vi "ActionVIOnCompile.vi"(8 "error in (no error)":errorcluster, 11 "Device Item Ref in":T1 format="%.0x") -> (0 "error out":errorcluster)   [LabVIEW 2016, in "UDP-Custom-Device System Explorer.lvlib"]
uses:
  UDP-Custom-Device System Explorer.lvlib
  <vilib>/NI Veristand/Custom Device API/Custom Device Item Ref.ctl
  Shared/Compiled.Settings.ctl
  Shared/Types/Shared - Rx.PacketInfo.ctl
  Shared/Types/Shared - Channel Data Type.ctl
  Shared/Types/Shared - Buffered.PacketInfo.ctl
  Shared/Types/Shared - Pointer Encoding.ctl
  Shared/Types/Shared - Receive Buffer Options.ctl
  Shared/Types/Shared - Transmit Buffer Options.ctl
  Shared/Types/Shared - Duplex Settings.ctl
  Shared/Types/Shared - New Data Options.ctl
  Shared/Types/Shared - Tx.PacketInfo.ctl
  Shared/Types/Shared - Transmit Flag Options.ctl
  Shared/Types/Shared - Transmit Echo Options.ctl
  Shared/Types/Shared - Transmit Sim Options.ctl
  Shared/Types/Shared - Header Details.ctl
  <vilib>/NI Veristand/Custom Device API/Set Item Property (Variant).vi
  <vilib>/NI VeriStand/Custom Device API/Custom Device API.lvlib
  <vilib>/NI/NIVS Inline Async API/_Data Access System Explorer/Data Access System Explorer.lvlib
  Shared/UDP-Custom-Device Shared.lvlib
panel:
  out "appended array":T2(array[cluster]) {"VS Refs" format="%.0x"}
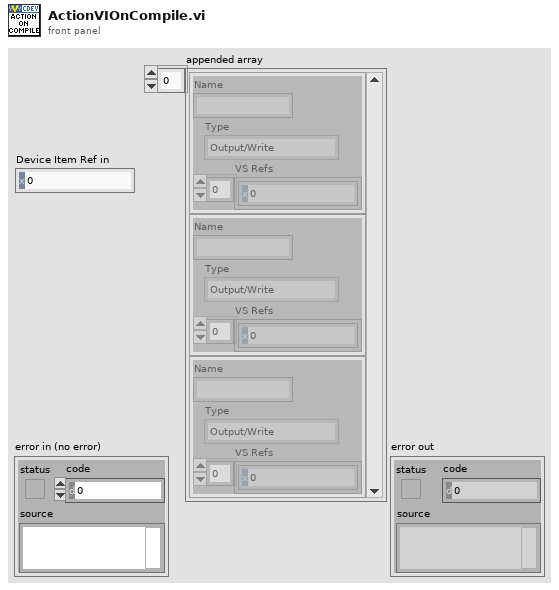
[diagram p1: front panel]
types:
  T1 = typedef "Custom Device API.lvlib/Custom Device Item Ref.ctl" = u64
  T2 = cluster{"Name":string, "Type":enum16{"Output/Write", "Input/Read", "Input/ReadWrite"}, "VS Refs":T1[]}[]
  T3 = typedef "UDP-Custom-Device Shared.lvlib/Compiled.Settings.ctl" = cluster{"Name":string, "Tx Enabled?":bool, "Rx Enabled?":bool, "Rx Packet Info":T4[], "Tx Packet Info":T11[], "Duplex Packets":refnum<data-value>}
  T4 = typedef "UDP-Custom-Device Shared.lvlib/Shared - Rx.PacketInfo.ctl" = cluster{"Packet Name":string, "Packet ID":i32, "Timeout":i32, "Rx IP Address":string, "Rx Port":u16, "Endianness":u16, "Multicast":bool, "Multicast IP Address":string, "Diagnostics En?":bool, "Debug Mode":bool, "Header Info":bool[], "Channel Data Types":T5[], "Buffered Packet Info":T6, "Duplex Packets":refnum<data-value>, "New Data Option":T10, "targetPriority":i16, "targetProcessor":i8}
  T5 = typedef "UDP-Custom-Device Shared.lvlib/Shared - Channel Data Type.ctl" = enum16{"Boolean", "Single", "Double", "I8", "I16", "I32", "I64", "U8", "U16", "U32", "U64"}
  T6 = typedef "UDP-Custom-Device Shared.lvlib/Shared - Buffered.PacketInfo.ctl" = cluster{"Buffer Size":i32, "External Buffer":bool, "Prepend Header":bool, "Is Buffered":bool, "Pointer Encoding":T7, "Rx Buffer Option":T8, "Tx Buffer Option":T9}
  T7 = typedef "UDP-Custom-Device Shared.lvlib/Shared - Pointer Encoding.ctl" = enum16{"Direct Encoding", "Conversion Encoding"}
  T8 = typedef "UDP-Custom-Device Shared.lvlib/Shared - Receive Buffer Options.ctl" = enum16{"Static Buffer", "Circular Buffer", "Circular Buffer + Size"}
  T9 = typedef "UDP-Custom-Device Shared.lvlib/Shared - Transmit Buffer Options.ctl" = enum16{"Static Buffer", "FIFO Buffer", "FIFO Buffer + Port"}
  T10 = typedef "UDP-Custom-Device Shared.lvlib/Shared - New Data Options.ctl" = enum16{"Timeout Reset", "Counter"}
  T11 = typedef "UDP-Custom-Device Shared.lvlib/Shared - Tx.PacketInfo.ctl" = cluster{"Packet Name":string, "Packet ID":i32, "Decimation":u16, "Destination IP Address":string, "Destination Port":u16, "Local IP Address":string, "Local Port":u16, "Endianness":u16, "TTL":u16, "Multicast":bool, "Multicast IP Address":string, "Transmit Option":T12, "Transmit Echo Option":T13, "Transmit Sim Option":T14, "Port as Channel":bool, "Debug Mode":bool, "Header Info":bool[], "Loop Period":u32, "Channel Data Types":T5[], "Header Details":T15, "Buffered Packet Info":T6, "Duplex Packets":refnum<data-value>, "targetProcessor":i8, "targetPriority":i16}
  T12 = typedef "UDP-Custom-Device Shared.lvlib/Shared - Transmit Flag Options.ctl" = enum16{"Always", "One-Shot", "Toggle"}
  T13 = typedef "UDP-Custom-Device Shared.lvlib/Shared - Transmit Echo Options.ctl" = enum16{"PCL Reset", "Counter", "Mirror"}
  T14 = typedef "UDP-Custom-Device Shared.lvlib/Shared - Transmit Sim Options.ctl" = enum16{"No Simulation", "Counter", "Full Buffer", "FIFO Test", "FIFO + Port Test"}
  T15 = typedef "UDP-Custom-Device Shared.lvlib/Shared - Header Details.ctl" = cluster{"Packet Size":u16, "Protocol Revision":u8, "System Definition Version":u64, "Source Node Name":string, "Packet ID":u32, "Number of Channels":u32, "Static Header Size":u16, "Total Header Size":u16}
  T16 = typedef "Custom Device API.lvlib/Custom Device Item Info.ctl" = cluster{"Name":string, "Is Channel":bool, "GUID":string, "Is Waveform":bool}
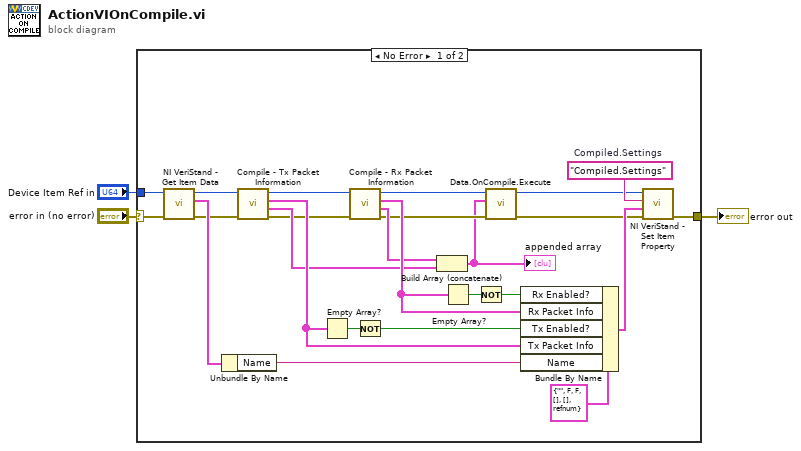
[diagram p0: block diagram]
diagram:
  n1 = case shown="No Error" "error in (no error)" {
    selector: "error in (no error)" -> [w26 w29]
    tunnel: [w27 w29] -> w2
    tunnel: "Device Item Ref in" -> [w25 _]
    frame No Error {
      w28 = "Compiled.Settings"  # Compiled.Settings
      n2 = call <vilib>:"NI VeriStand - Get Item Data.vi"("error in (no error)"=w26, "Item Ref in"=w25) -> ("error out"=w11:errorcluster, "Item Info"=w24:T16, "Item Ref out"=w12:T1)  [unwired: 6 in, 1 out]
      n3 = Unbundle By Name(w24) -> ("Name"=w19:string)
      n4 = call "Compile - Tx Packet Information.vi"("error in (no error)"=w11, "Custom Device Ref in"=w12) -> ("error out"=w8:errorcluster, "Tx Ref Array"=w14:T2, "Tx Packet Info Array"=w15:T11[], "Custom Device Ref out"=w10:T1)  [unwired: 6 in]
      n5 = Empty Array?(array=w15) -> (empty?=w21:bool)
      n6 = call "Compile - Rx Packet Information.vi"("error in (no error)"=w8, "Custom Device Ref in"=w10) -> ("error out"=w6:errorcluster, "Rx Ref Array"=w13:T2, "Rx Packet Info Array"=w16:T4[], "Custom Device Ref out"=w9:T1)  [unwired: 6 in]
      n7 = Not(x=w21) -> (.not. x?=w17:bool)
      n8 = Build Array (concatenate)(w13, w14) -> (w5:T2)
      "appended array" <- w5
      n9 = Empty Array?(array=w16) -> (empty?=w20:bool)
      n10 = Not(x=w20) -> (.not. x?=w18:bool)
      n11 = call <vilib>:"Data.OnCompile.Execute.vi"("error in"=w6, "VS Ref Groups"=w5, "Custom Device Ref"=w9) -> ("error out"=w4:errorcluster, "Custom Device Ref"=w22:T1)  [unwired: 7 in]
      n12 = Bundle By Name(cluster=T3 {"Name"="", "Tx Enabled?"=FALSE, "Rx Enabled?"=FALSE, "Rx Packet Info"=[], "Tx Packet Info"=[], "Duplex Packets"=refnum} ("Compiled.Settings"), "Rx Enabled?"=w18, "Rx Packet Info"=w16, "Tx Enabled?"=w17, "Tx Packet Info"=w15, "Name"=w19) -> (w7:T3)
      n13 = call-poly <vilib>:"NI VeriStand - Set Item Property.vi"("error in (no error)"=w4, "Value"=w7, "Property Name"=w28, "Item Ref in"=w22) -> ("error out"=w27:errorcluster)  [unwired: 5 in, 2 out]
    }
    frame Error {
    }
  }
  "error out" <- w2
